vi "Handle Command.vi"(8 "error in":errorcluster, 10 "Load New Speaker Chirp in":refnum<class "Load New Speaker Chirp.lvclass">, 11 "Object In":refnum<class>) -> (0 "error out":errorcluster, 1 "Command Successful?":bool, 2 "Load New Speaker Chirp Out":refnum<class "Load New Speaker Chirp.lvclass">, 3 "Object Out":refnum<class>)   [LabVIEW 2018, in "ePAS Library.lvlib" / "Load New Speaker Chirp.lvclass"]
doc: "Load a new speaker tophat. The tophat is a broadband \"chirp\" that allows the caller to characterize te acoustic properties of the cavity (retrieve Q and f0)."
uses:
  Load New Speaker Chirp.lvclass
  Instrument/ePAS.lvclass
  C:/Users/Labview/Documents/exscalabar_server/reusable/PAS/Main/PAS.lvclass
  C:/Users/Labview/Documents/exscalabar_server/reusable/Instrument/Instrument.lvclass
  FPGA/Session/Exscalabar FPGA.lvclass
  Instrument/ePAS.lvclass/ePAS.ctl
  Load New Speaker Chirp.lvclass/Load New Speaker Chirp.ctl
  reusable/PAS/Main/PAS.lvclass/PAS.ctl
  reusable/Instrument/Instrument.lvclass/Instrument.ctl
  FPGA/Session/Exscalabar FPGA.lvclass/Exscalabar FPGA.ctl
  FPGA/Session/Read Ex FPGA Ref.vi
  reusable/Instrument/Read Log Session.vi
  <vilib>/Utility/error.llb/Error Cluster From Error Code.vi
  <vilib>/rvi/errors/niLvFpgaAdjustHostInterfaceError.vi
  FPGA/R FPGA Ref.ctl
  <vilib>/rvi/interface/nirviMethod/nirviMethod.xnode
  FPGA Bitfiles/FPGAServer.lvbitx
  <userlib>/_Session Fwk/Session - Root.lvclass
  reusable/PAS/Main/PAS.lvclass
  ePAS Library.lvlib
  reusable/Session APIs/Session Log/System Log.lvclass
  <vilib>/FPGAPlugInAG/PXI-7842R/niLvFpga_WriteFifo_PXI-7842R.vi
  <vilib>/rvi/errors/niLvFpgaMergeErrorWithErrorCode.vi
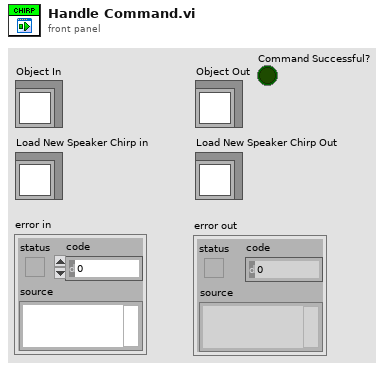
[diagram p1: front panel]
types:
  T1 = typedef "Session - Root.lvclass/Session Handle.ctl" = refnum<data-value>
  T2 = typedef "ePAS Library.lvlib/R FPGA Ref.ctl" = refnum<k20>
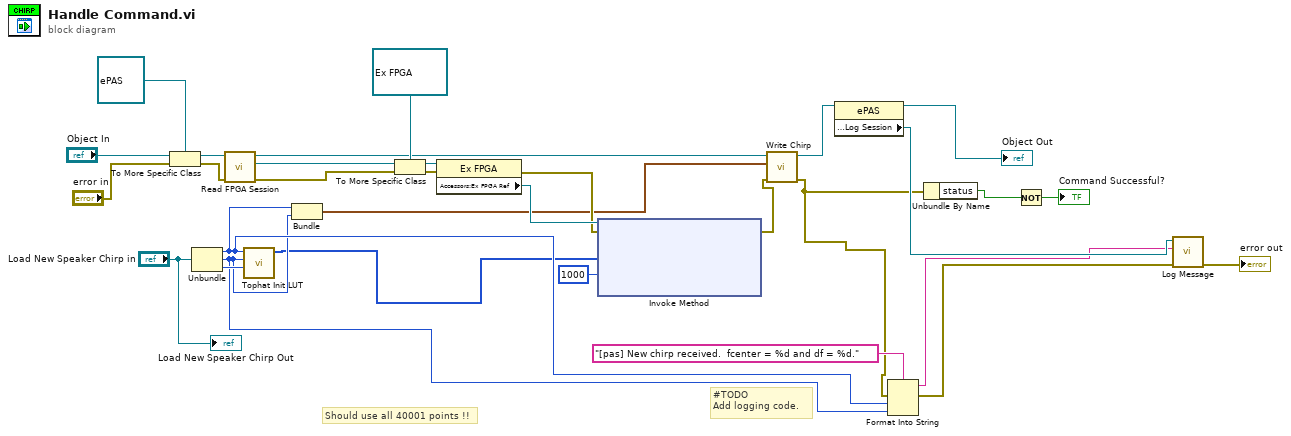
[diagram p0: block diagram]
diagram:
  # "Should use all 40001 points !!"
  # "#TODO\nAdd logging code."
  n1 = To More Specific Class(target class=refnum<class "ePAS.lvclass"> refnum ("ePAS.lvclass"), reference="Object In", error in="error in") -> (specific class reference=w28:refnum<class "ePAS.lvclass">, error out=w18:errorcluster)
  n2 = Unbundle("Load New Speaker Chirp in") -> (w7:i16, w6:i16, w31:i32)
  n3 = call "Read FPGA Session.vi"("error in (no error)"=w18, "ePAS in"=w28) -> ("error out"=w20:errorcluster, "Session Handle"=w26:T1, "ePAS out"=w17:refnum<class "ePAS.lvclass">)  [unwired: 7 in]
  n4 = call "Tophat Init LUT.vi"("Number of  Elements"=w31, "Df"=w6, "f0"=w7) -> ("Init Data Out"=w1:i16[])  [unwired: 6 in]
  n5 = Bundle("fcenter"=w7, "bandwidth"=w6) -> (w15:cluster{"fcenter":i16, "bandwidth":i16})  [unwired: 1 in]
  n6 = To More Specific Class(target class=refnum<data-value> refnum ("Session Handle"), reference=w26, error in=w20) -> (specific class reference=w24:refnum<data-value>, error out=w23:errorcluster)
  n7 = property class="Ex FPGA"(reference=w24, error in=w23) -> (error out=w19:errorcluster, "Accessors:Ex FPGA Ref"=w22:T2)  [unwired: 1 out]
  n8 = xnode "Invoke Method"("FPGA VI Reference In"=w22, "error in"=w19, "Data"=w1, "Timeout (ms)"=1000) -> ("error out"=w16:errorcluster)  [unwired: 2 out]
  n9 = call "Write Chirp.vi"("error in (no error)"=w16, "Chirp"=w15, "PAS in"=w17) -> ("error out"=w4:errorcluster, "PAS out"=w11:refnum<class "ePAS.lvclass">)  [unwired: 7 in]
  n10 = property class="ePAS"(reference=w11) -> (reference out=→"Object Out":refnum<class "ePAS.lvclass">, "Accessors:Log Session"=w10:T1)  [unwired: 1 in, 1 out]
  n11 = Format Into String(format string="[pas] New chirp received.  fcenter = %d and df = %d.", error in=w4, w7, w6) -> (resulting string=w5:string, error out=w3:errorcluster)  [unwired: 1 in]
  n12 = Unbundle By Name(w4) -> ("status"=w13:bool)
  n13 = Not(x=w13) -> (.not. x?=→"Command Successful?":bool)
  n14 = call "Log Message.vi"("error in"=w3, "MSG In"=w5, "session in"=w10) -> ("error out"=→"error out":errorcluster)  [unwired: 7 in, 1 out]
  "Load New Speaker Chirp Out" <- "Load New Speaker Chirp in"
